vi "publisher tests Reader 9.vi"() -> ()   [LabVIEW 2018]
uses:
  publisher action.ctl
panel:
  out "number":dbl
  in  "read":bool
  out "Numeric":i32
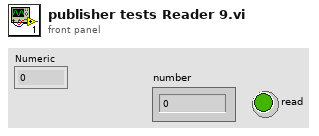
[diagram p1: front panel]
types:
  T1 = typedef "publisher action.ctl" = enum16{"set", "get", "init", "check"}
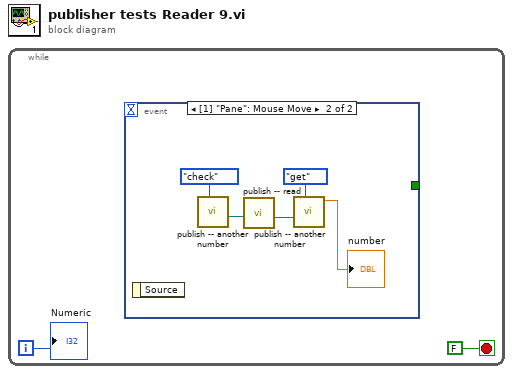
[diagram p0: block diagram]
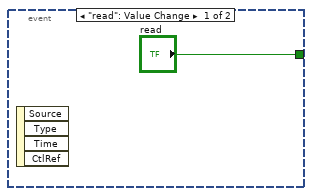
[diagram p2: hidden frame]
diagram:
  n1 = while {
    i -> [w1]
    stop <- FALSE stop-if-true
    n2 = event shown="[1] \"Pane\": Mouse Move" {
      selector: _ -> [_ _]
      dyn-events: _ -> [_ _]
      timeout: _ -> [_ _]
      tunnel: ["read" _] -> _
      event "read": Value Change {
        n3 = event-data() -> ()  [unwired: 1 in, 4 out]
      }
      event Mouse Move {
        n4 = event-data() -> ()  [unwired: 1 in, 1 out]
        n5 = call "publish -- another number.vi"("publisher action"=publisher_action."check") -> ("recieve event"=w7:refnum<user-event>)  [unwired: 8 in, 2 out]
        n6 = call "publish -- read.vi"("recieve event"=w7) -> ("recieve event OUT"=w6:refnum<user-event>)  [unwired: 10 in]
        n7 = call "publish -- another number.vi"("publisher action"=publisher_action."get", "recieve event inn"=w6) -> ("Numeric out"=→"number":dbl)  [unwired: 7 in, 2 out]
      }
    }
    "Numeric" <- w1
  }
